vi "GetStreamingFilter.vi"(8 "error in (no error)":errorcluster, 11 "Ref in":T4) -> (0 "error out":errorcluster, 2 "IDs":T1, 3 "Ref out":T4)   [LabVIEW 2019, in "Protection and Counter Host Automation API.lvlib"]
uses:
  Protection and Counter Host Automation API.lvlib
  Types/API Variables.ctl
  <vilib>/NI/STM/TCP/TCP Connection Info.ctl
  <vilib>/NI/STM/SubVIs/MetaDataElement.ctl
  SubModules/CAN-Streaming-Support/Source/Addon/Addon Shared/Types/Filter Parameters.ctl
  SubModules/CAN-Streaming-Support/Source/Addon/Addon Shared/Types/Direction Filter.ctl
  SubModules/CAN-Streaming-Support/Source/Addon/Addon Shared/Types/Type Filter.ctl
  <vilib>/NI/NI VeriStand Addon Network Comm/Shared/NI VeriStand Addon Network Comm Shared.lvlib
  SubModules/CAN-Streaming-Support/Source/Addon/Addon Shared/CAN Stream Support Shared.lvlib
  <vilib>/NI/STM/NI STM.lvlib
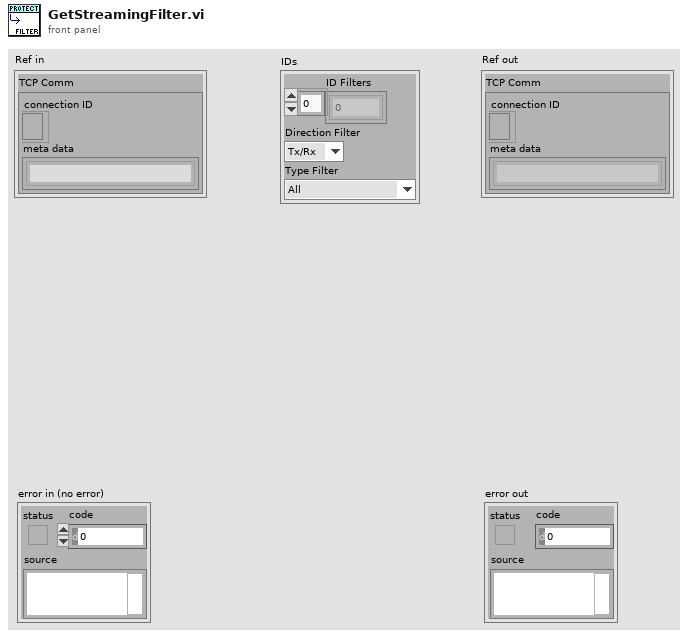
[diagram p1: front panel]
types:
  T1 = typedef "CAN Stream Support Shared.lvlib/Filter Parameters.ctl" = cluster{"ID Filters":u32[], "Direction Filter":T2, "Type Filter":T3}
  T2 = typedef "CAN Stream Support Shared.lvlib/Direction Filter.ctl" = enum16{"Tx/Rx", "Rx", "Tx"}
  T3 = typedef "CAN Stream Support Shared.lvlib/Type Filter.ctl" = enum16{"All", "CAN Data", "CAN Remote", "CAN Bus Error", "CAN 2.0 Data", "CAN FD Data", "CAN FD+BRS Data", "J1939 Data", "Delay", "Log Trigger", "Start Trigger"}
  T4 = typedef "Protection and Counter Host Automation API.lvlib/API Variables.ctl" = cluster{"TCP Comm":T5}
  T5 = typedef "NI STM.lvlib/TCP Connection Info.ctl" = cluster{"connection ID":refnum<k5>, "meta data":T6[]}
  T6 = typedef "NI STM.lvlib/MetaDataElement.ctl" = string
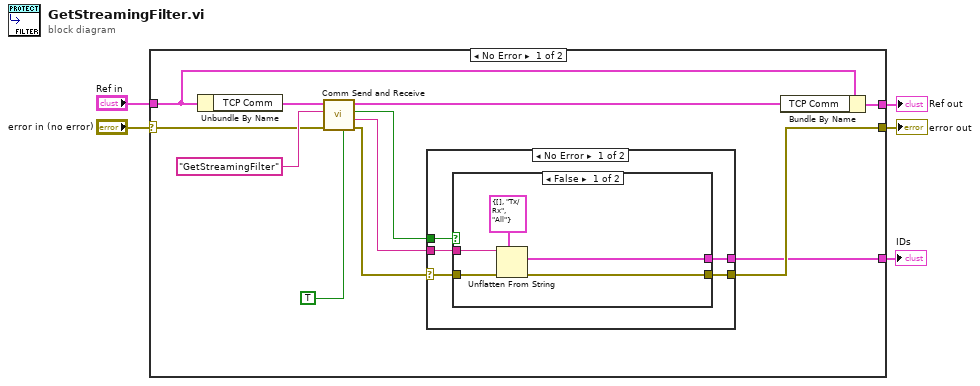
[diagram p0: block diagram]
diagram:
  n1 = case shown="No Error" "error in (no error)" {
    selector: "error in (no error)" -> [w7 w31]
    tunnel: "Ref in" -> [w15 w30]
    tunnel: [w13 w30] -> w4
    tunnel: [w9 w31] -> w3
    tunnel: [w6 _] -> w1
    frame No Error {
      n2 = Unbundle By Name(w15) -> ("TCP Comm"=w16:T5)
      n3 = call <vilib>:"Comm Send and Receive.vi"("Resp Required?"=TRUE, "error in (no error)"=w7, "Name"="GetStreamingFilter", "connection info"=w16) -> ("error out"=w10:errorcluster, "Data"=w12:string, "Timed Out?"=w11:bool, "connection info"=w14:T5)  [unwired: 4 in]
      n4 = case shown="No Error" w10 {
        selector: w10 -> [w20 w29]
        tunnel: w11 -> [w22 _]
        tunnel: [w21 w29] -> w9
        tunnel: w12 -> [w19 _]
        tunnel: [w18 _] -> w6
        frame No Error {
          n5 = case shown="False" w22 {
            tunnel: [w26 w28] -> w21
            tunnel: w20 -> [w27 w28]
            tunnel: w19 -> [w25 _]
            tunnel: [w24 _] -> w18
            frame False {
              n6 = Unflatten From String(type=T1 {"ID Filters"=[], "Direction Filter"=enum."Tx/Rx", "Type Filter"=enum."All"} ("IDs"), binary string=w25, error in (no error)=w27) -> (value=w24:T1, error out=w26:errorcluster)  [unwired: 2 in, 1 out]
            }
            frame True {
            }
          }
        }
        frame Error {
        }
      }
      n7 = Bundle By Name(cluster=w15, "TCP Comm"=w14) -> (w13:T4)
    }
    frame Error {
    }
  }
  "Ref out" <- w4
  "error out" <- w3
  "IDs" <- w1
